vi "Turret_Set.vi"   [LabVIEW 2019]
uses:
  Turret_Globals.vi
types:
  T1 = enum16{"Manual_PercentVoltage", "Manual_SpeedControl", "Auto_Targeting"}
  T2 = typedef "Turret_Cluster.ctl" = cluster{"Control_State":enum16{"Manual_PercentVoltage", "Manual_SpeedControl", "Auto_Targeting"}, "Spin_Power":dbl, "Flywheel_Power":dbl}
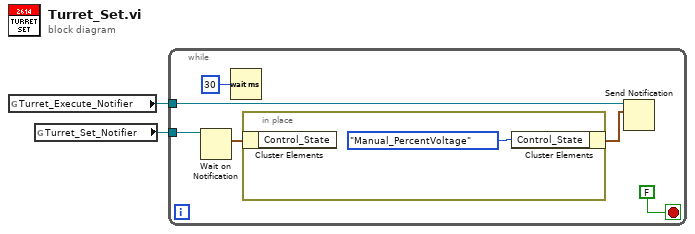
[diagram p0: block diagram]
diagram:
  n1 = global read "Turret_Globals.vi" "Turret_Execute_Notifier"() -> (w1:refnum<notifier>)
  n2 = global read "Turret_Globals.vi" "Turret_Set_Notifier"() -> (w2:refnum<notifier>)
  n3 = while {
    tunnel: w2 -> [w6]
    tunnel: w1 -> [w3]
    stop <- FALSE stop-if-true
    n4 = Wait on Notification(notifier=w6) -> (notification=w5:T2)  [unwired: 3 in, 3 out]
    n5 = Wait (ms)(milliseconds to wait=u32 30) -> ()  [unwired: 1 out]
    n6 = in-place {
      n7 = in-place-cluster #1(w5) -> ()  [unwired: 1 out]
      n8 = in-place-cluster #1("Control_State"=T1."Manual_PercentVoltage") -> (w4:T2)
    }
    n9 = Send Notification(notification=w4, notifier=w3) -> ()  [unwired: 1 in, 2 out]
  }
